vi "OnCollision.vi"(7 "Game in":refnum<class "Game.lvclass">, 8 "error in (no error)":errorcluster, 9 "Engine in":refnum<class "Engine.lvclass">, 10 "Collider":refnum<class "GameObject.lvclass">, 11 "GameObject in":refnum<class "GameObject.lvclass">) -> (0 "error out":errorcluster, 1 "Engine out":refnum<class "Engine.lvclass">, 2 "Colliderout":refnum<class "GameObject.lvclass">, 3 "GameObject out":refnum<class "GameObject.lvclass">, 5 "Game out":refnum<class "Game.lvclass">)   [LabVIEW 2019, in "RT_Game.lvlib" / "GameObject.lvclass"]
uses:
  GameObject.lvclass
  Game/Game.lvclass
  Engine/Engine.lvclass
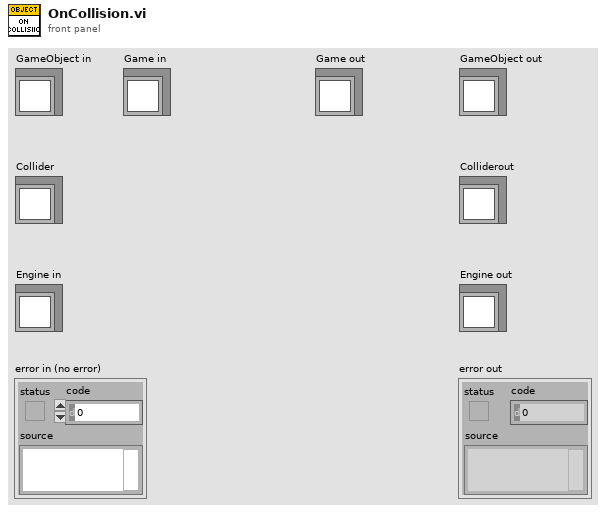
[diagram p1: front panel]
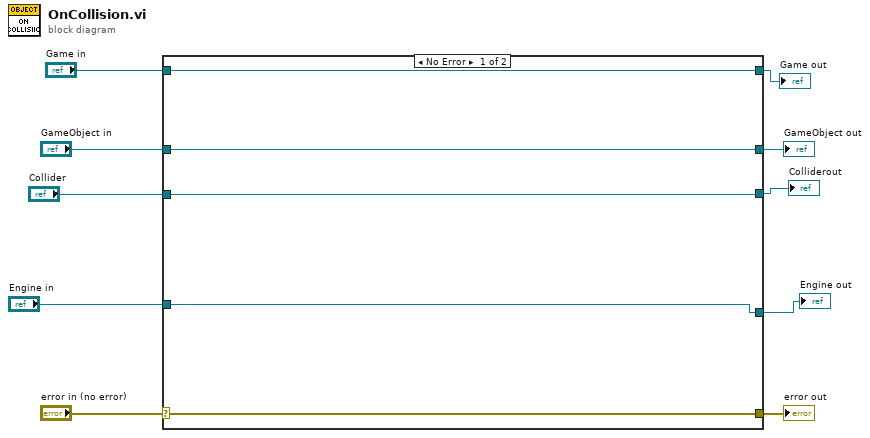
[diagram p0: block diagram]
diagram:
  n1 = case shown="No Error" "error in (no error)" {
    selector: "error in (no error)" -> [w14 w20]
    tunnel: [w14 w20] -> w9
    tunnel: [w15 w19] -> w7
    tunnel: "GameObject in" -> [w15 w19]
    tunnel: [w13 w18] -> w5
    tunnel: "Collider" -> [w13 w18]
    tunnel: [w12 w17] -> w4
    tunnel: "Game in" -> [w12 w17]
    tunnel: [w11 w16] -> w2
    tunnel: "Engine in" -> [w11 w16]
    frame No Error {
    }
    frame Error {
    }
  }
  "error out" <- w9
  "GameObject out" <- w7
  "Colliderout" <- w5
  "Game out" <- w4
  "Engine out" <- w2
